vi "Get Controller Card Model.vi"(8 "error in (no error)":errorcluster, 11 "controllerCardModel":string) -> (0 "error out":errorcluster, 2 "function return":u32, 3 "controllerCardModel out":string)   [LabVIEW 2014, in "atmcd32d.lvlib"]
doc: "unsigned int WINAPI GetControllerCardModel(char * controllerCardModel);"
uses:
  atmcd32d.lvlib
  atmcd32d.dll
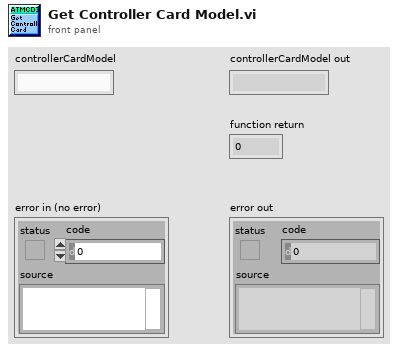
[diagram p1: front panel]
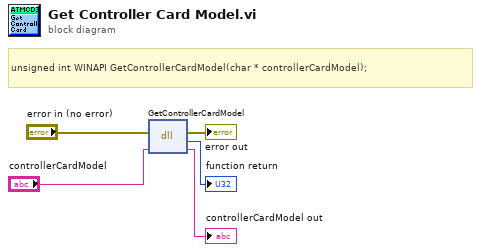
[diagram p0: block diagram]
diagram:
  # "unsigned int WINAPI GetControllerCardModel(char * controllerCardModel);"
  n1 = dll-call lib="C:/Users/Bakir/Documents/Lambda2-Testing/lib/Andorlib/atmcd32d.*" fn="GetControllerCardModel"(error in="error in (no error)", "controllerCardModel"="controllerCardModel") -> (error out=→"error out":errorcluster, →"function return":u32, "controllerCardModel"=→"controllerCardModel out":string)  [unwired: 2 in, 1 out]
